vi "SpiralPoints.vi"(0 "m: Number of spirals/turn":u16=36 min=1, 1 "a: Pitch (turns smaller than width)":dbl=44.0, 2 "r0: Start Radius":dbl=2000.0, 3 "width (radius)":dbl=2000.0, 4 "Track density (1= equal in xy)":dbl=1.0 min=1e-06) -> (5 "Coordinates":cdb[](array[numeric]), 6 "imax: number of points per spiral":u32=541)   [LabVIEW 2011]
panel:
  out "XY Graph":cluster{dbl, dbl}[](graph)
  # "Pattern is Yoko-type\noption calulate pitch from n points\nsee SpiralPoints-FixedPoints.vi"
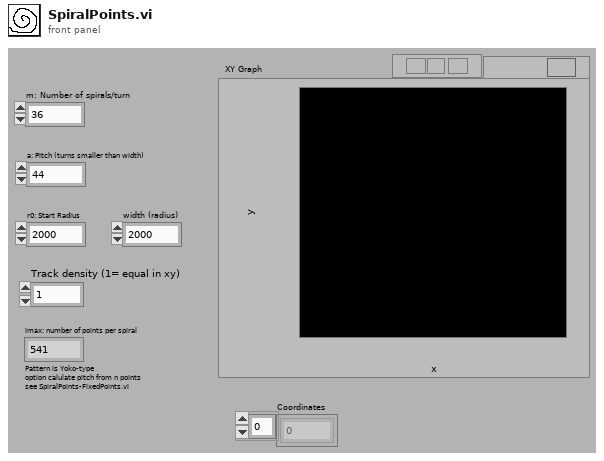
[diagram p1: front panel]
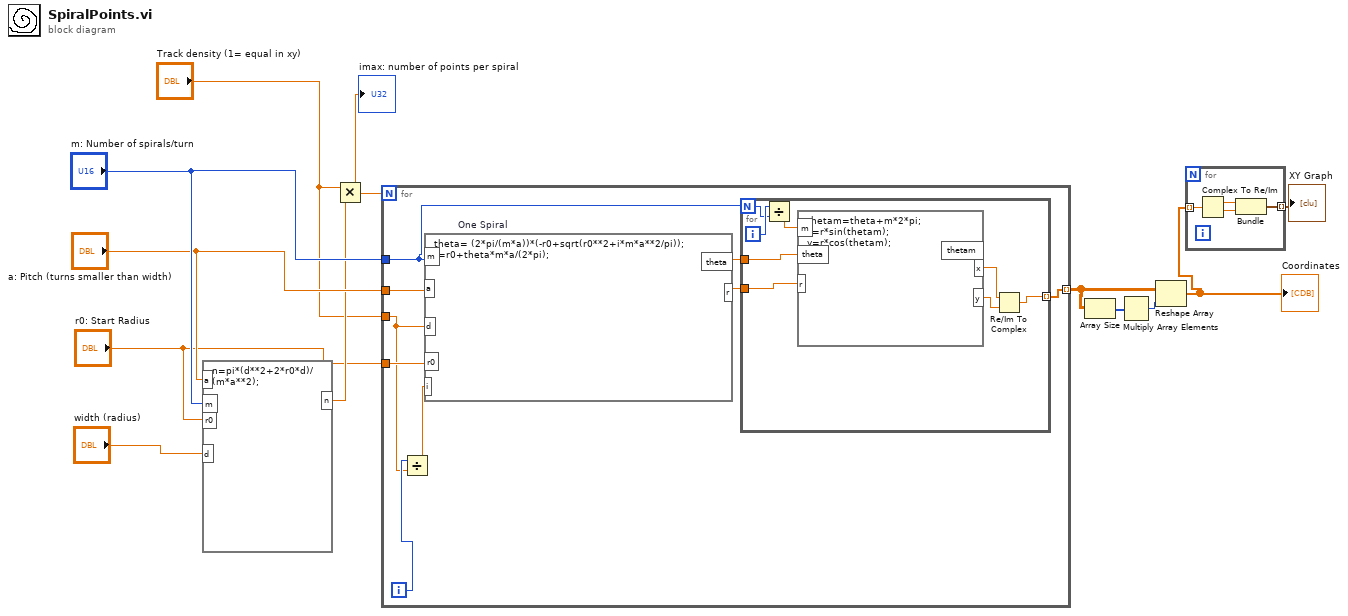
[diagram p0: block diagram]
diagram:
  n1 = formula code="n=pi*(d**2+2*r0*d)/(m*a**2);"("r0"="r0: Start Radius", "d"="width (radius)", "a"="a: Pitch (turns smaller than width)", "m"="m: Number of spirals/turn") -> ("n"=w7:dbl)
  n2 = Multiply(x="Track density (1= equal in xy)", y=w7) -> (x*y=w2:dbl)
  "imax: number of points per spiral" <- w2
  n3 = for {
    N: w2 -> [_]
    tunnel: "m: Number of spirals/turn" -> [w17]
    tunnel: "a: Pitch (turns smaller than width)" -> [w21]
    tunnel: "r0: Start Radius" -> [w20]
    tunnel: [w16] -> w12 mode=indexing
    tunnel: "Track density (1= equal in xy)" -> [w13]
    i -> [w14]
    n4 = Divide(x=w14, y=w13) -> (x/y=w15:dbl)
    n5 = formula code="theta= (2*pi/(m*a))*(-r0+sqrt(r0**2+i*m*a**2/pi));\nr=r0+theta*m*a/(2*pi);" "One Spiral"("m"=w17, "a"=w21, "i"=w15, "r0"=w20, "d"=w13) -> ("theta"=w19:dbl, "r"=w18:dbl)
    n6 = for {
      N: w17 -> [w27]
      tunnel: [w22] -> w16 mode=indexing
      tunnel: w19 -> [w29]
      tunnel: w18 -> [w25]
      i -> [w28]
      n7 = Divide(x=w28, y=w27) -> (x/y=w26:dbl)
      n8 = formula code="thetam=theta+m*2*pi;\nx=r*sin(thetam);\ny=r*cos(thetam);"("theta"=w29, "r"=w25, "m"=w26) -> ("x"=w24:dbl, "y"=w23:dbl)  [unwired: 1 out]
      n9 = Re/Im To Complex(1:w23, 2:w24) -> (0:w22:cdb)
    }
  }
  n10 = Array Size(array=w12) -> (size(s)=w10:i32[])
  n11 = Multiply Array Elements(1:w10) -> (0:w11:i32)
  n12 = Reshape Array(w12, w11) -> (w4:cdb[])
  "Coordinates" <- w4
  n13 = for {
    tunnel: w4 -> [w33] mode=indexing
    tunnel: [w30] -> w3 mode=indexing
    n14 = Complex To Re/Im(x + iy=w33) -> (x=w32:dbl, y=w31:dbl)
    n15 = Bundle(w32, w31) -> (w30:cluster{dbl, dbl})  [unwired: 1 out]
  }
  "XY Graph" <- w3
